vi "api_mqttPublish.vi"(0 "topic":string, 5 "value":string, 7 "QoS (At most once)":T3, 9 "messageID":u16, 11 "error in (no error)":errorcluster, 12 "retain(F)":bool, 13 "duplicate(F)":bool) -> (4 "success":bool, 15 "error out":errorcluster)   [LabVIEW 2022 SP3, in "mqtt.lvclass"]
uses:
  mqtt.lvclass
  mqttTypedef/mqttQOSlevel.ctl
  mqttTypedef/mqttRXdataCluster.ctl
  mqttTypedef/mqttFixedHeaderResponse.ctl
  mqttTypedef/mqttMessageType.ctl
  mqttCmd/mqttCmdPublish/mqttCmdPublish.lvclass
  D:/Mac study folder/2022Fall/3CC3/_2022CCFinal/SRA_labview_ubidots/class/mqtt/mqttCmd/mqttCmd.lvclass
  mqttCmd/mqttCmdPublish/mqttCmdPublish.lvclass/mqttCmdPublish.ctl
  mqttCmd/mqttCmd.lvclass/mqttCmd.ctl
  mqttCmd/mqttCmd.lvclass
panel:
  out "notification":T1
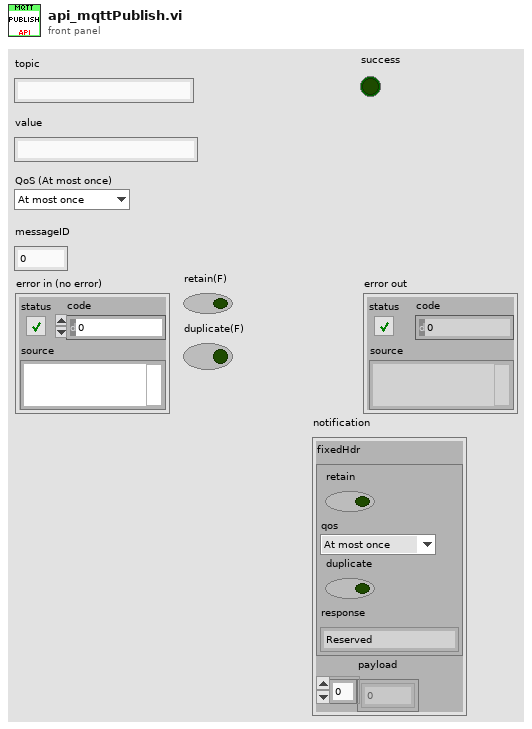
[diagram p1: front panel]
types:
  T1 = typedef "mqttRXdataCluster.ctl" = cluster{"fixedHdr":T2, "payload":u8[]}
  T2 = typedef "mqttFixedHeaderResponse.ctl" = cluster{"retain":bool, "qos":T3, "duplicate":bool, "response":T4}
  T3 = typedef "mqttQOSlevel.ctl" = enum8{"At most once", "At least once", "Exactly once", "Reserved"}
  T4 = typedef "mqttMessageType.ctl" = enum32{"Reserved", "CONNECT", "CONNACK", "PUBLISH", "PUBACK", "PUBREC", "PUBREL", "PUBCOMP", "SUBSCRIBE", "SUBACK", "UNSUBSCRIBE", "UNSUBACK", "PINGREQ", "PINGRESP", "DISCONNECT", "Reserved2"}
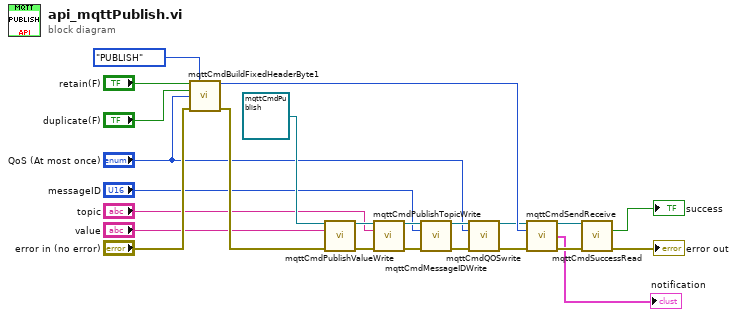
[diagram p0: block diagram]
diagram:
  n1 = call "mqttCmdBuildFixedHeaderByte1.vi"("retain(F)"="retain(F)", "MessageType"=mqttMessageType."PUBLISH", "duplicate(F)"="duplicate(F)", "QoS (At most once)"="QoS (At most once)", "error in (no error)"="error in (no error)") -> ("byte1"=w23:u8, "error out"=w19:errorcluster)  [unwired: 9 in]
  n2 = call "mqttCmdPublishValueWrite.vi"("mqttPublish in"=refnum<class "mqttCmdPublish.lvclass"> refnum ("mqttPublish.lvclass"), "value"="value", "error in (no error)"=w19) -> ("mqttPublish out"=w16:refnum<class "mqttCmdPublish.lvclass">, "error out"=w18:errorcluster)  [unwired: 11 in]
  n3 = call "mqttCmdPublishTopicWrite.vi"("mqttPublish in"=w16, "topic"="topic", "error in (no error)"=w18) -> ("mqttPublish out"=w10:refnum<class "mqttCmdPublish.lvclass">, "error out"=w11:errorcluster)  [unwired: 11 in]
  n4 = call "mqttCmdMessageIDWrite.vi"("mqttBrokerCommand in"=w10, "messageID"="messageID", "error in (no error)"=w11) -> ("mqttBrokerCommand out"=w6:refnum<class "mqttCmdPublish.lvclass">, "error out"=w8:errorcluster)  [unwired: 11 in]
  n5 = call "mqttCmdQOSwrite.vi"("mqttBrokerCommand in"=w6, "QoS"="QoS (At most once)", "error in (no error)"=w8) -> ("mqttBrokerCommand out"=w5:refnum<class "mqttCmdPublish.lvclass">, "error out"=w7:errorcluster)  [unwired: 11 in]
  n6 = call "mqttCmdSendReceive.vi"("mqttConnect in"=w5, "byte1"=w23, "error in (no error)"=w7) -> ("mqttConnect out"=w3:refnum<class "mqttCmdPublish.lvclass">, "notification"=→"notification":T1, "error out"=w2:errorcluster)  [unwired: 10 in]
  n7 = call "mqttCmdSuccessRead.vi"("mqttBrokerCommand in"=w3, "error in (no error)"=w2) -> ("success"=→"success":bool, "error out"=→"error out":errorcluster)  [unwired: 11 in, 1 out]
